vi "get_exp_from_groupSD.vi"(3 "error in (no error)":errorcluster, 4 "group":u16, 5 "exp selected":i32, 6 "Experiments groups":refnum<class "Experiments_group.lvclass">[](array[class])) -> (0 "error out":errorcluster, 1 "Group":refnum<class "Experiments_group.lvclass">, 2 "Experiment out":refnum<class "Experiment.lvclass">)   [LabVIEW 2015]
uses:
  Classes/Experiment.lvclass
  Classes/Experiments_group.lvclass
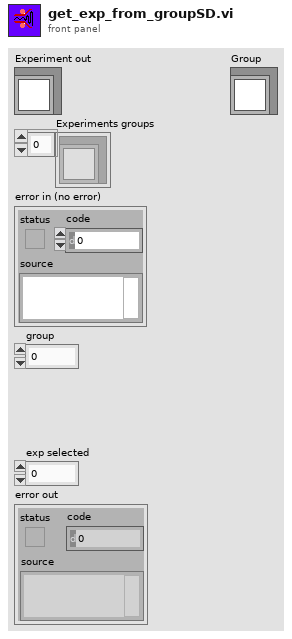
[diagram p1: front panel]
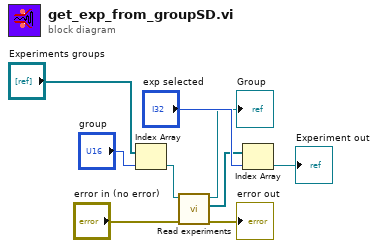
[diagram p0: block diagram]
diagram:
  n1 = Index Array(array="Experiments groups", index="group") -> (element=w2:refnum<class "Experiments_group.lvclass">)
  n2 = call "Read experiments.vi"("error in (no error)"="error in (no error)", "Experiments_group.lvclass in"=w2) -> ("error out"=→"error out":errorcluster, "Experiments"=w3:refnum<class "Experiment.lvclass">[], "Experiments_group.lvclass out"=→"Group":refnum<class "Experiments_group.lvclass">)  [unwired: 6 in]
  n3 = Index Array(array=w3, index="exp selected") -> (element=→"Experiment out":refnum<class "Experiment.lvclass">)
